vi "Substitute Panel VI.vi"(7 "VI Reference":refnum<vi>, 10 "SubPanel Reference":refnum<vi>) -> (0 "error out":errorcluster)   [LabVIEW 2016, in "Assert API Components.lvlib" / "Assert Display.lvlib" / "Base UI Component.lvlib" / "Base UI Component.lvclass"]
uses:
  Base UI Component.lvclass
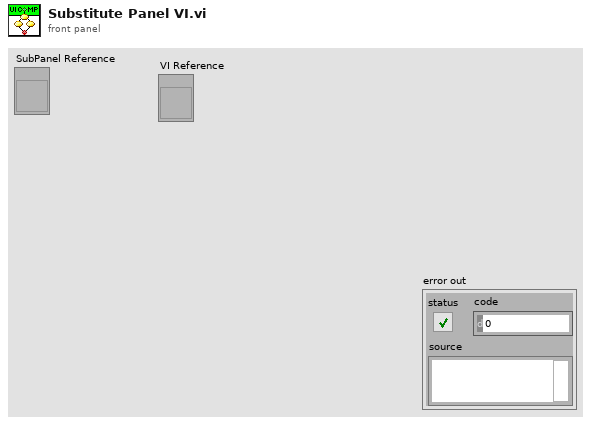
[diagram p1: front panel]
types:
  T1 = enum32{"Invalid", "Standard", "Closed", "Hidden", "Minimized", "Maximized"}
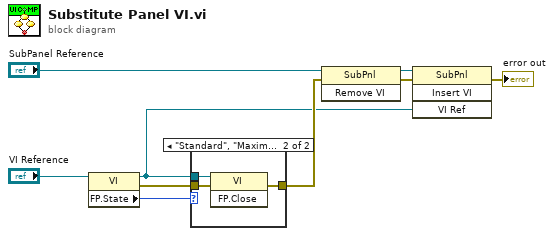
[diagram p0: block diagram]
diagram:
  n1 = property class="VI"(reference="VI Reference") -> (reference out=w1:refnum<vi>, error out=w3:errorcluster, "FP.State"=w2:T1)  [unwired: 1 in]
  n2 = case shown="\"Standard\", \"Maximized\"" w2 {
    tunnel: [w10 w13] -> w4
    tunnel: w1 -> [_ w12]
    tunnel: w3 -> [w10 w11]
    frame Default {
    }
    frame "Standard", "Maximized" {
      n3 = invoke class="VI" method="FP.Close"(reference=w12, error in=w11) -> (error out=w13:errorcluster)  [unwired: 1 in, 2 out]
    }
  }
  n4 = invoke class="SubPnl" method="Remove VI"(reference="SubPanel Reference", error in=w4) -> (reference out=w9:refnum<vi>, error out=w8:errorcluster)  [unwired: 1 in, 1 out]
  n5 = invoke class="SubPnl" method="Insert VI"(reference=w9, error in=w8, "VI Ref"=w1) -> (error out=→"error out":errorcluster)  [unwired: 1 in, 3 out]
